vi "tcsWEP_logEvent_comcamTargetWfsList.vi"(8 "error in (no error)":errorcluster, 11 "logevent_comcamTargetWfsList_Ctl":T1={"sensorIdList[9]"=[0, 0, 0, 0, 0, 0, 0, 0, 0], "timestamp"=0.0, "priority"=0}) -> (0 "error out":errorcluster, 2 "function return":i32, 3 "logevent_comcamTargetWfsList_Ctl out":T1)   [LabVIEW 2016, in "SALLV_tcsWEP.lvlib"]
doc: "int tcsWEP_shm_logEvent_comcamTargetWfsListLV(tcsWEP_logevent_comcamTargetWfsListLV *logevent_comcamTargetWfsList_Ctl );"
uses:
  SALLV_tcsWEP.lvlib
  DataTypes/logevent_comcamTargetWfsList.ctl
  SALLV_tcsWEP.so
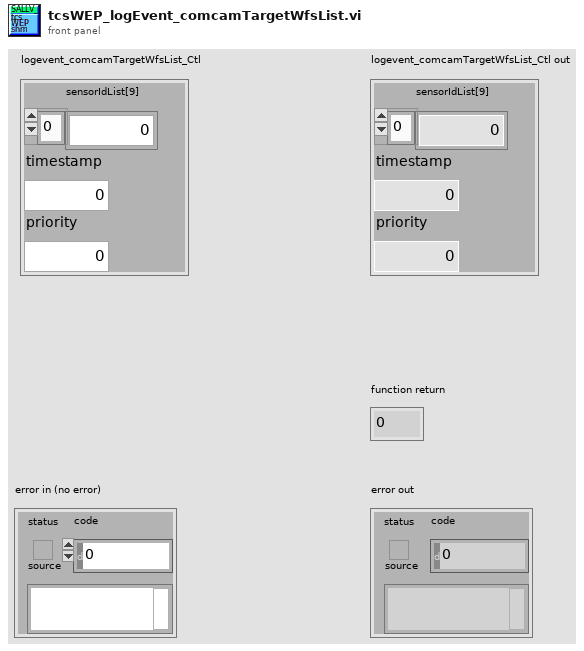
[diagram p1: front panel]
types:
  T1 = typedef "SALLV_tcsWEP.lvlib/logevent_comcamTargetWfsList.ctl" = cluster{"sensorIdList[9]":i16[], "timestamp":dbl, "priority":i32}
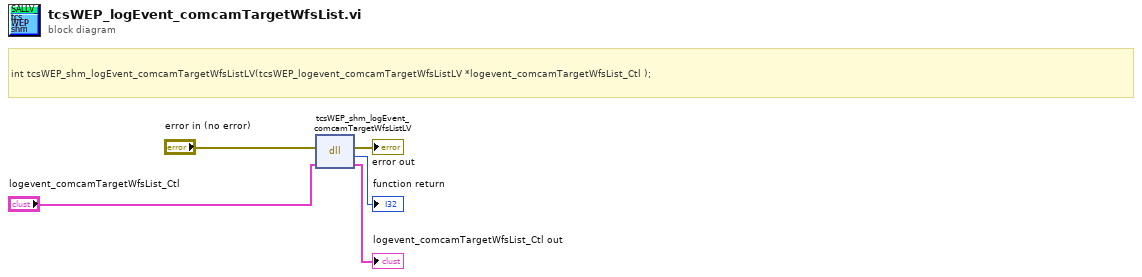
[diagram p0: block diagram]
diagram:
  # "int tcsWEP_shm_logEvent_comcamTargetWfsListLV(tcsWEP_logevent_comcamTargetWfsListLV *logevent_comcamTargetWfsList_Ctl );"
  n1 = dll-call lib="home/ttsai/Documents/salAPI/SALLV_tcsWEP.*" fn="tcsWEP_shm_logEvent_comcamTargetWfsListLV"(error in="error in (no error)", "logevent_comcamTargetWfsList_Ctl"="logevent_comcamTargetWfsList_Ctl") -> (error out=→"error out":errorcluster, →"function return":i32, "logevent_comcamTargetWfsList_Ctl"=→"logevent_comcamTargetWfsList_Ctl out":T1)  [unwired: 2 in, 1 out]
